vi "OM3_PostStimCleaning.vi"   [LabVIEW 2015]
uses:
  Intrinsic Rig/software/widefield_imaging_OM2/control_VIs/OM2_control_VIs/global_cleaning_0621.vi
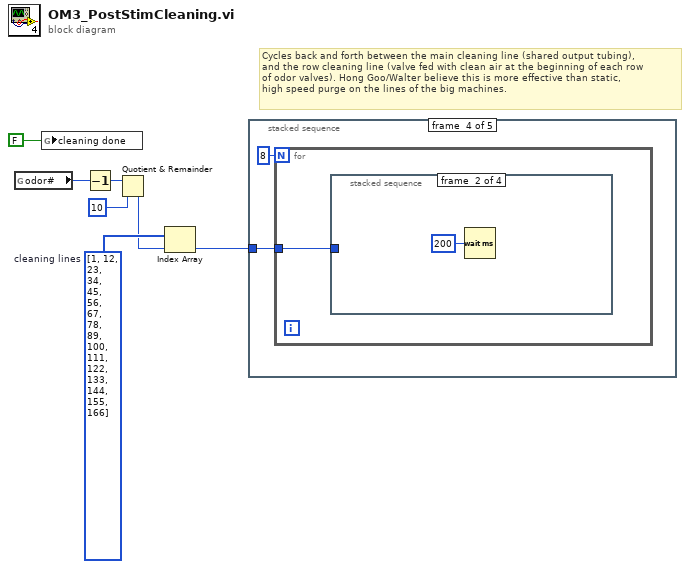
[diagram p0: block diagram]
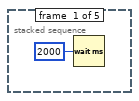
[diagram p2: hidden frame]
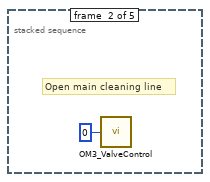
[diagram p3: hidden frame]
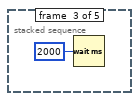
[diagram p4: hidden frame]
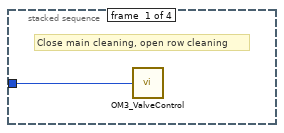
[diagram p5: hidden frame]
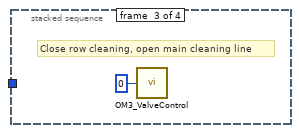
[diagram p6: hidden frame]
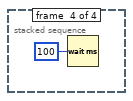
[diagram p7: hidden frame]
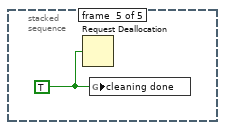
[diagram p8: hidden frame]
diagram:
  w7 = i32[] [1, 12, 23, 34, 45, 56, 67, 78, 89, 100, 111, 122, 133, 144, 155, 166]  # cleaning lines
  # "Cycles back and forth between the main cleaning line (shared output tubing),\nand the row cleaning line (valve fed with clean air at the beginning of each row \nof odor valves). Hong Goo/Walter believe this is more effective than static, \nhigh speed purge on the lines of the big machines."
  n1 = global read "global_cleaning_0621.vi" "odor#"() -> (w2:i32)
  n2 = global write "global_cleaning_0621.vi" "cleaning done"(FALSE ("cleaning done")) -> ()
  n3 = Decrement(x=w2) -> (x-1=w4:i32)
  n4 = Quotient & Remainder(x=w4, y=10) -> (floor(x/y)=w6:i32)  [unwired: 1 out]
  n5 = Index Array(array=w7, index=w6) -> (element=w1:i32)
  n6 = stacked-sequence {
    tunnel: w1 -> [_ _ _ w12 _]
    frame #0 {
      n7 = Wait (ms)(milliseconds to wait=u32 2000) -> ()  [unwired: 1 out]
    }
    frame #1 {
      # "Open main cleaning line"
      n8 = call "OM3_ValveControl.vi"("Valve#"=0) -> ()  [unwired: 1 in]
    }
    frame #2 {
      n9 = Wait (ms)(milliseconds to wait=u32 2000) -> ()  [unwired: 1 out]
    }
    frame #3 {
      n10 = for {
        N: 8 -> [_]
        tunnel: w12 -> [w13]
        n11 = stacked-sequence {
          tunnel: w13 -> [w14 _ _ _]
          frame #0 {
            # "Close main cleaning, open row cleaning"
            n12 = call "OM3_ValveControl.vi"("Valve#"=w14) -> ()  [unwired: 1 in]
          }
          frame #1 {
            n13 = Wait (ms)(milliseconds to wait=u32 200) -> ()  [unwired: 1 out]
          }
          frame #2 {
            # "Close row cleaning, open main cleaning line"
            n14 = call "OM3_ValveControl.vi"("Valve#"=0) -> ()  [unwired: 1 in]
          }
          frame #3 {
            n15 = Wait (ms)(milliseconds to wait=u32 100) -> ()  [unwired: 1 out]
          }
        }
      }
    }
    frame #4 {
      w18 = TRUE ("cleaning done")
      n16 = Request Deallocation(w18) -> ()
      n17 = global write "global_cleaning_0621.vi" "cleaning done"(w18) -> ()
    }
  }
